vi "Teleop - Intake Control.vi"(10 "Buttons 2":bool[](array[boolean]), 11 "Buttons":bool[](array[boolean])) -> ()   [LabVIEW 2017]
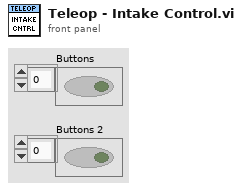
[diagram p1: front panel]
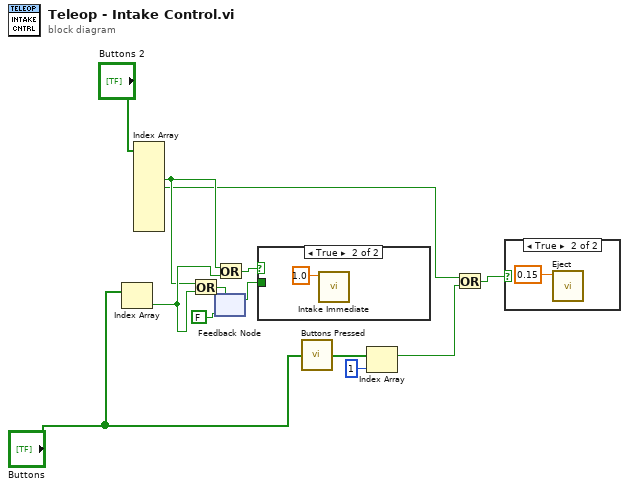
[diagram p0: block diagram]
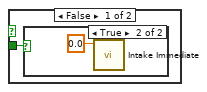
[diagram p3: hidden frame]
diagram:
  n1 = Index Array(array="Buttons") -> (element=w8:bool)  [unwired: 1 in]
  n2 = Index Array(array="Buttons 2") -> (element #3=w7:bool, element #4=w5:bool)  [unwired: 9 in, 7 out]
  n3 = Or(x=w7, y=w8) -> (x .or. y?=w6:bool)
  n4 = feedback #1(FALSE) -> (w1:bool)
  n5 = feedback-in #1(w6) -> ()
  n6 = Or(x=w7, y=w8) -> (x .or. y?=w3:bool)
  n7 = case shown="True" w3 {
    tunnel: w1 -> [w14 _]
    frame False {
      n8 = case shown="True" w14 {
        frame False {
        }
        frame True {
          n9 = call "Intake Immediate.vi"("Setpoint"=0.0) -> ()  [unwired: 10 in, 1 out]
        }
      }
    }
    frame True {
      n10 = call "Intake Immediate.vi"("Setpoint"=1.0) -> ()  [unwired: 10 in, 1 out]
    }
  }
  n11 = call "Buttons Pressed.vi"("Button Values"="Buttons") -> ("Button Presses"=w11:bool[])
  n12 = Index Array(array=w11, index=1) -> (element=w12:bool)
  n13 = Or(x=w5, y=w12) -> (x .or. y?=w4:bool)
  n14 = case shown="True" w4 {
    frame False {
    }
    frame True {
      n15 = call "Eject.vi"("Setpoint"=0.15 ("Eject Power")) -> ()  [unwired: 10 in, 1 out]
    }
  }
